vi "AlliGator Find Cross-Correlation Shift.vi"(4 "normalization (none)":enum32{"none", "unbiased", "biased"}(ring)=enum."unbiased", 5 "polynomial order (3)":i32=3, 6 "Reference Decay":cluster{"t Array":dbl[], "I Array":dbl[]}, 7 "Half Width (Points)":i32=5 min=3, 8 "Error In":errorcluster, 9 "Time Stamp":dbl, 10 "Lifetime Graph":refnum<vi>, 11 "Decay Graph":refnum<vi>) -> (0 "Error Out":errorcluster, 3 "Zero Position":dbl)   [LabVIEW 2021, in "AlliGator Decay Preprocessing.lvlib"]
doc: "Computes the shift of the last plot in the <B>Decay Graph</B> maximizing the cross-correlation of that plot and the <B>Reference Decay</b> and adds this value to the last plot in the <B>Lifetime & Other Parameters Graph</b>."
uses:
  AlliGator Decay Preprocessing.lvlib
  Graphs/XY Graph/XY Graph Add-Ons.lvlib
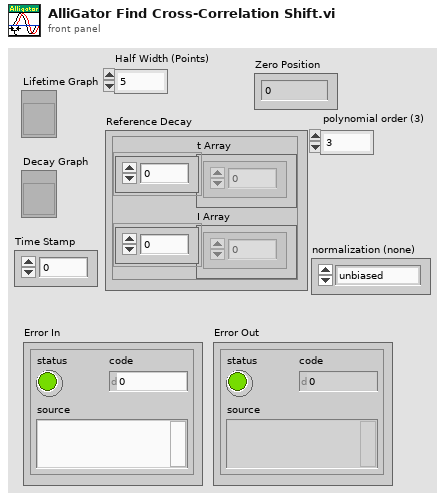
[diagram p1: front panel]
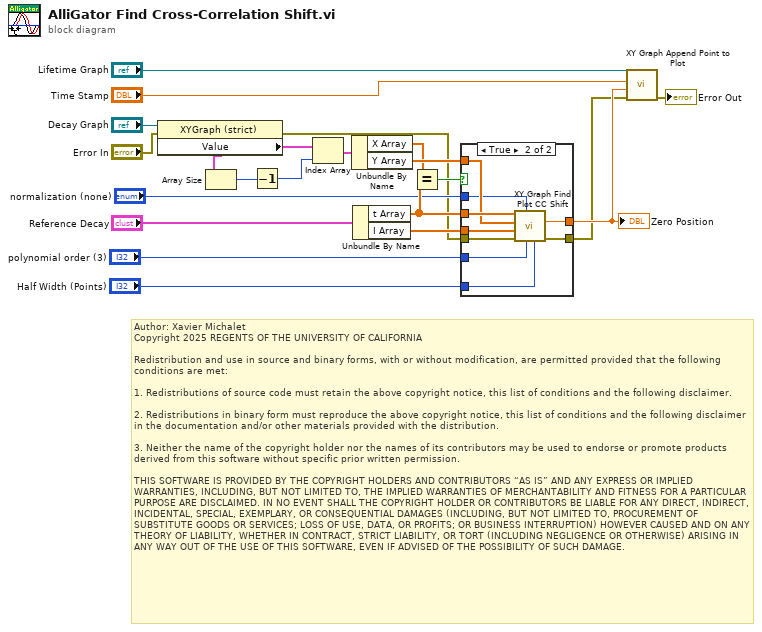
[diagram p0: block diagram]
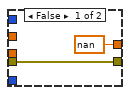
[diagram p2: hidden frame]
diagram:
  # "Author: Xavier Michalet\nCopyright 2025 REGENTS OF THE UNIVERSITY OF CALIFORNIA\n\nRedistribution and use in source and binary forms, with or without modification, are permitted provided that the following conditions are met:\n\n1. Redistributions of source code must retain the above copyright notice, this list of conditions and the following disclaimer.\n\n2. Redistributions in binary form must reproduce the above copyright notice, this list of conditions and the following disclaimer in the documentation and/or other materials provided with the distribution.\n\n3. Neither the name of the copyright holder nor the names of its contributors may be used to endorse or promote products derived from this software without specific prior written permission.\n\nTHIS SOFTWARE IS PROVIDED BY THE COPYRIGHT HOLDERS AND CONTRIBUTORS “AS IS” AND ANY EXPRESS OR IMPLIED WARRANTIES, INCLUDING, BUT NOT LIMITED TO, THE IMPLIED WARRANTIES OF MERCHANTABILITY AND FITNESS FOR A PARTICULAR PURPOSE ARE DISCLAIMED. IN NO EVENT SHALL THE COPYRIGHT HOLDER OR CONTRIBUTORS BE LIABLE FOR ANY DIRECT, INDIRECT, INCIDENTAL, SPECIAL, EXEMPLARY, OR CONSEQUENTIAL DAMAGES (INCLUDING, BUT NOT LIMITED TO, PROCUREMENT OF SUBSTITUTE GOODS OR SERVICES; LOSS OF USE, DATA, OR PROFITS; OR BUSINESS INTERRUPTION) HOWEVER CAUSED AND ON ANY THEORY OF LIABILITY, WHETHER IN CONTRACT, STRICT LIABILITY, OR TORT (INCLUDING NEGLIGENCE OR OTHERWISE) ARISING IN ANY WAY OUT OF THE USE OF THIS SOFTWARE, EVEN IF ADVISED OF THE POSSIBILITY OF SUCH DAMAGE."
  n1 = property class="XYGraph (strict)"(reference="Decay Graph", error in="Error In") -> (error out=w2:errorcluster, "Value"=w19:cluster{"X Array":dbl[], "Y Array":dbl[]}[])  [unwired: 1 out]
  n2 = Array Size(array=w19) -> (size(s)=w18:i32)
  n3 = Decrement(x=w18) -> (x-1=w14:i32)
  n4 = Index Array(array=w19, index=w14) -> (element=w17:cluster{"X Array":dbl[], "Y Array":dbl[]})
  n5 = Unbundle By Name(w17) -> ("X Array"=w10:dbl[], "Y Array"=w12:dbl[])
  n6 = Unbundle By Name("Reference Decay") -> ("t Array"=w9:dbl[], "I Array"=w11:dbl[])
  n7 = Equal?(x=w10, y=w9) -> (x = y?=w3:bool)
  n8 = case shown="True" w3 {
    tunnel: w12 -> [_ w28]
    tunnel: w11 -> [_ w32]
    tunnel: w9 -> [_ w29]
    tunnel: [nan ("Shift") w31] -> w8
    tunnel: "Half Width (Points)" -> [_ w30]
    tunnel: "polynomial order (3)" -> [_ w25]
    tunnel: "normalization (none)" -> [_ w24]
    tunnel: w2 -> [w23 w27]
    tunnel: [w23 w26] -> w1
    frame False {
    }
    frame True {
      n9 = call "XY Graph Find Plot CC Shift.vi"("Half Width (Points)"=w30, "polynomial order"=w25, "normalization"=w24, "Error In"=w27, "Ref Array"=w32, "Y Array"=w28, "X Array"=w29) -> ("Error Out"=w26:errorcluster, "Shift"=w31:dbl)  [unwired: 2 in, 1 out]
    }
  }
  "Zero Position" <- w8
  n10 = call "XY Graph Append Point to Plot.vi"("error in (no error)"=w1, "y"=w8, "x"="Time Stamp", "XYGraph in"="Lifetime Graph") -> ("error out"=→"Error Out":errorcluster)  [unwired: 4 in, 3 out]
